vi "SmootherPath.vi"(6 "ball":T1, 8 "Robot in":T2={"id"=0, "function"=enum."Attacker", "x"=0.0, "y"=0.0, "orientation"=0.0, "v_tangent"=0.0, "v_normal"=0.0, "v_ang"=0.0, "kick_x"=0.0, "kick_z"=0.0, "dribble"=FALSE, "Timestamp"=timestamp(0 s since 1904-01-01), "estimatives"={"est_v_tangent"=0.0, "est_v_normal"=0.0, "est_vx"=0.0, "est_vy"=0.0, "Pos Robot Est"=[]}, "dest_x_kick"=0.0, "dest_y_kick"=0.0, "Gap Coord"=[], "States"=enum."GoToTangent", "Path "=[], "Path  Smooth"=[], "Dest"=[], "vx_desired"=0.0, "vy_desired"=0.0}, 9 "SmoothPath":dbl[][](array[numeric]), 10 "enemy_robots":T2[](array[typedef]), 11 "our_robots":T2[](array[typedef])) -> (1 "SmootherPath":dbl[][](array[numeric]))   [LabVIEW 2018]
uses:
  Vision_class/Old vision/Controls/AI Robot.ctl
  Vision_class/Old vision/Controls/Functions Enum.ctl
  Vision_class/Old vision/Controls/AttackerStates.ctl
  Vision_class/Old vision/Controls/PathDests.ctl
  Vision_class/Old vision/Controls/PathDest.ctl
  Communication_class/Paths/MessageAI_State Folder/Core/AI Ball.ctl
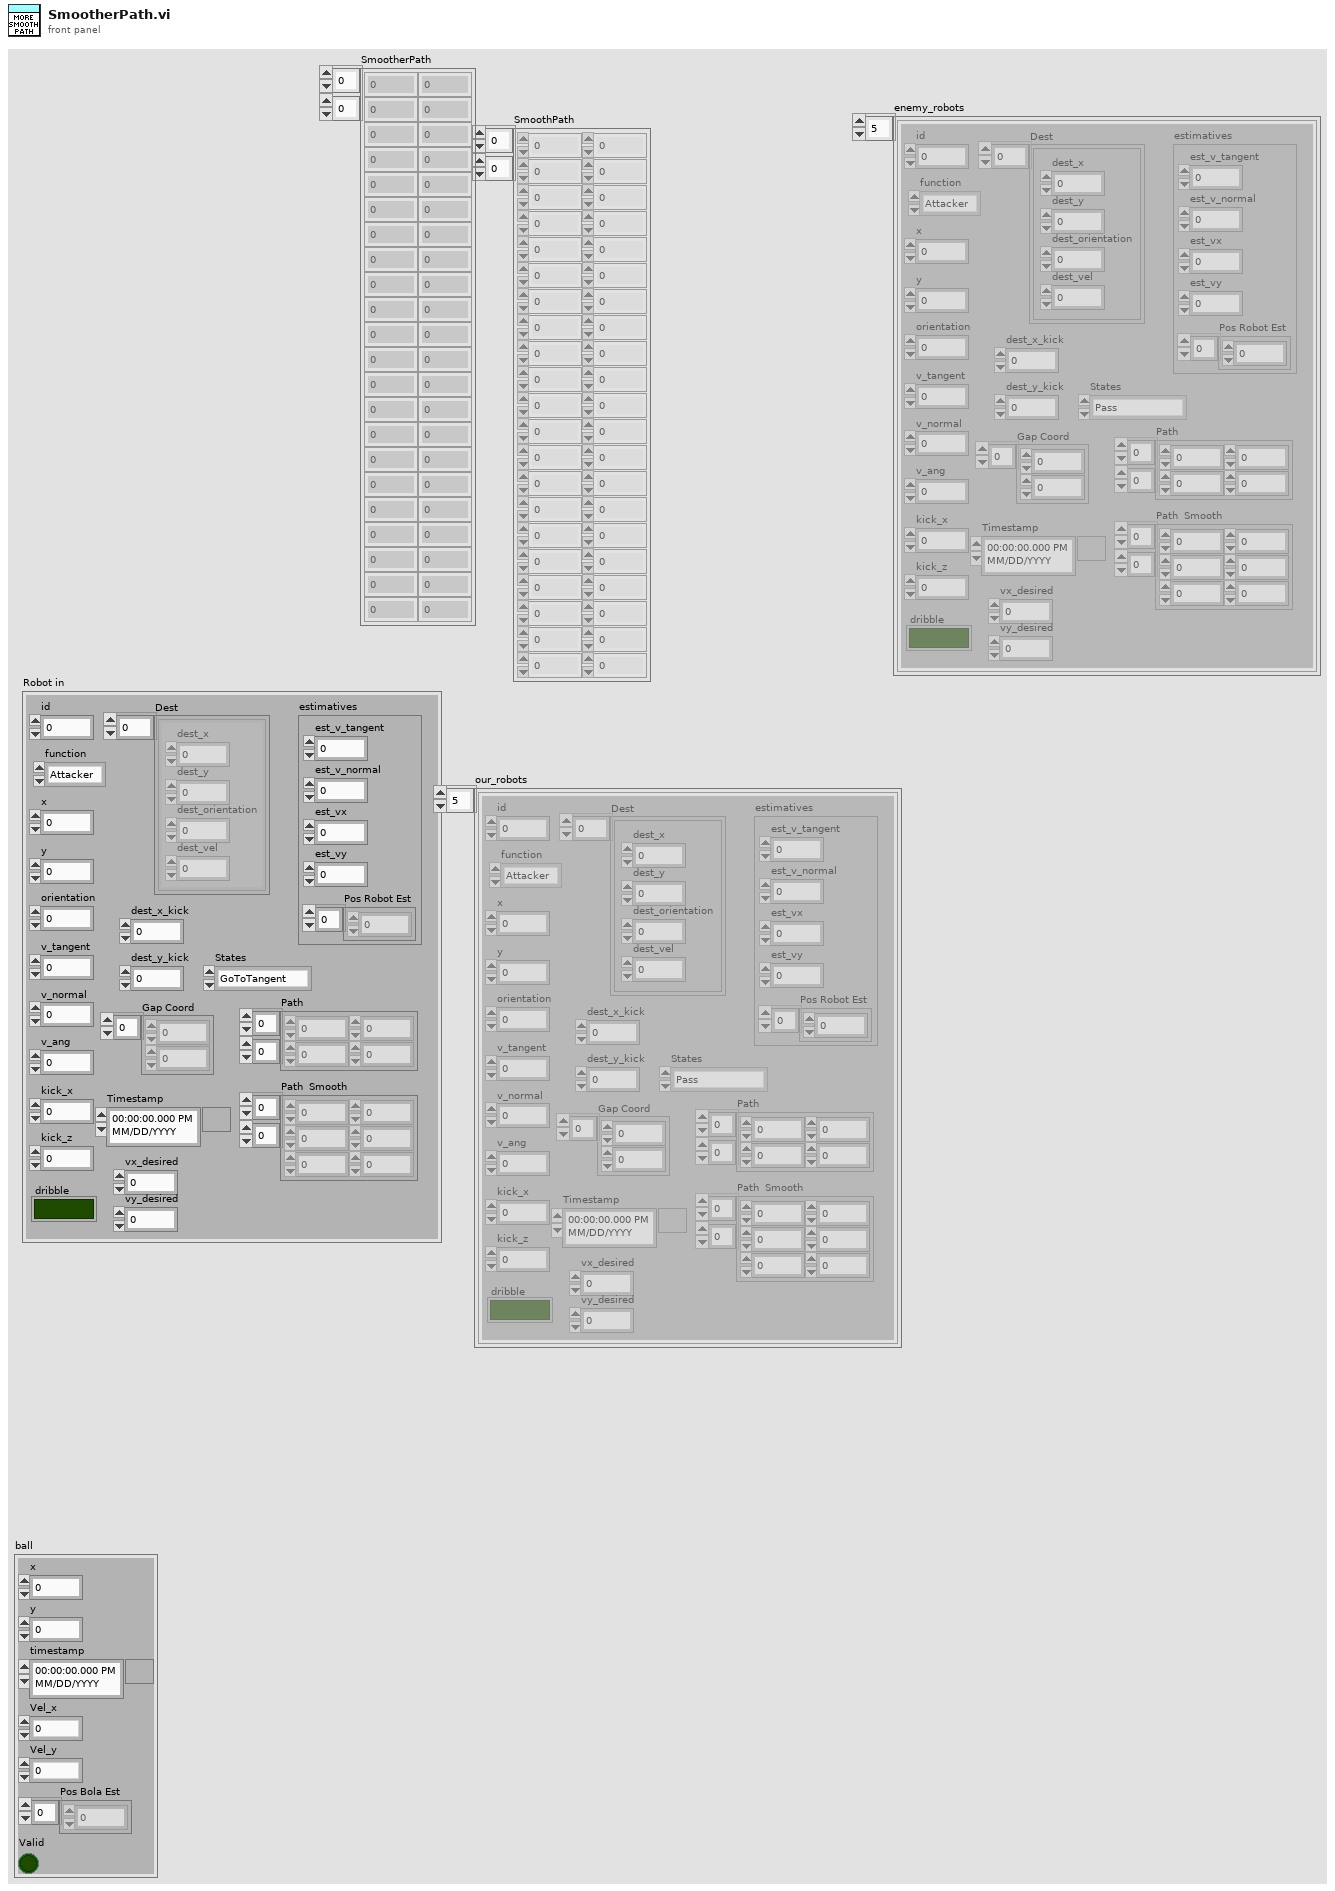
[diagram p1: front panel]
types:
  T1 = typedef "AI Ball.ctl" = cluster{"x":dbl, "y":dbl, "timestamp":timestamp, "Vel_x":dbl, "Vel_y":dbl, "Pos Bola Est":dbl[], "Valid":bool}
  T2 = typedef "AI Robot.ctl" = cluster{"id":u32, "function":T3, "x":dbl, "y":dbl, "orientation":dbl, "v_tangent":dbl, "v_normal":dbl, "v_ang":dbl, "kick_x":dbl, "kick_z":dbl, "dribble":bool, "Timestamp":timestamp, "estimatives":cluster{"est_v_tangent":dbl, "est_v_normal":dbl, "est_vx":dbl, "est_vy":dbl, "Pos Robot Est":dbl[]}, "dest_x_kick":dbl, "dest_y_kick":dbl, "Gap Coord":dbl[], "States":T4, "Path ":dbl[][], "Path  Smooth":dbl[][], "Dest":T5, "vx_desired":dbl, "vy_desired":dbl}
  T3 = typedef "Functions Enum.ctl" = enum16{"2nd Striker", "Attacker", "Goalie", "Defender", "Striker", "Goto 0", "Dummy", "Kicker", "ZigZag 0", "ZigZag 1", "ZigZag 2", "ZigZag 3", "ZigZag 4", "ZigZag 5", "ZigZag 6", "ZigZag 7", "ZigZag 8", ""}
  T4 = typedef "AttackerStates.ctl" = enum16{"Pass", "GoToTangent", "BallGetting", "GoToKick", ""}
  T5 = typedef "PathDests.ctl" = T6[]
  T6 = typedef "PathDest.ctl" = cluster{"dest_x":dbl, "dest_y":dbl, "dest_orientation":dbl, "dest_vel":dbl}
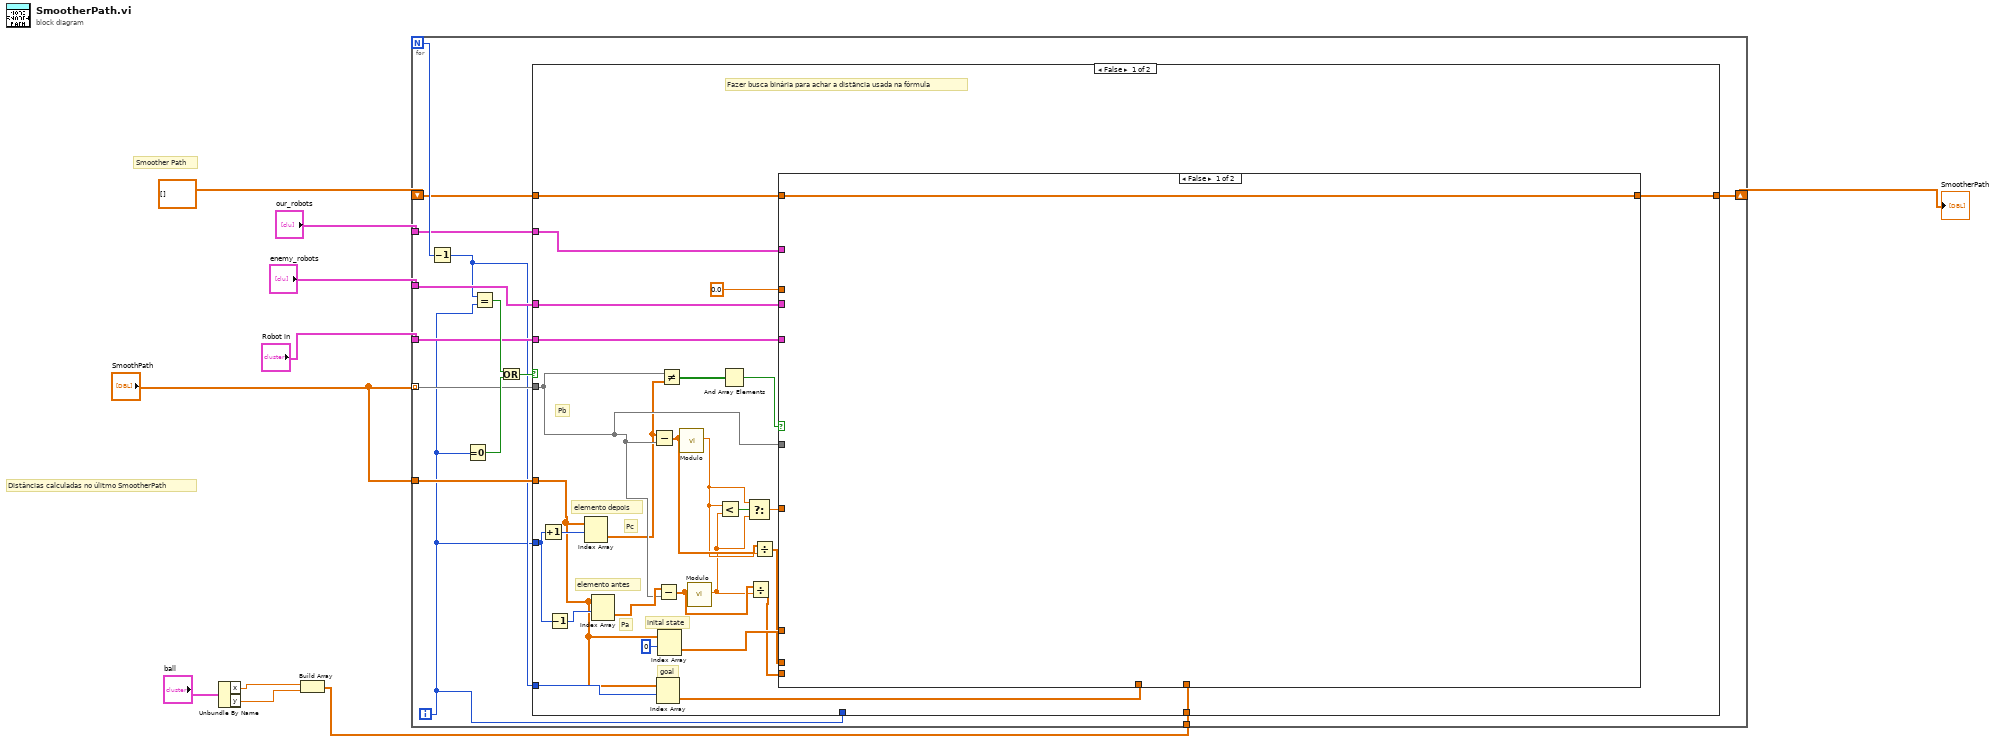
[diagram p0: block diagram]
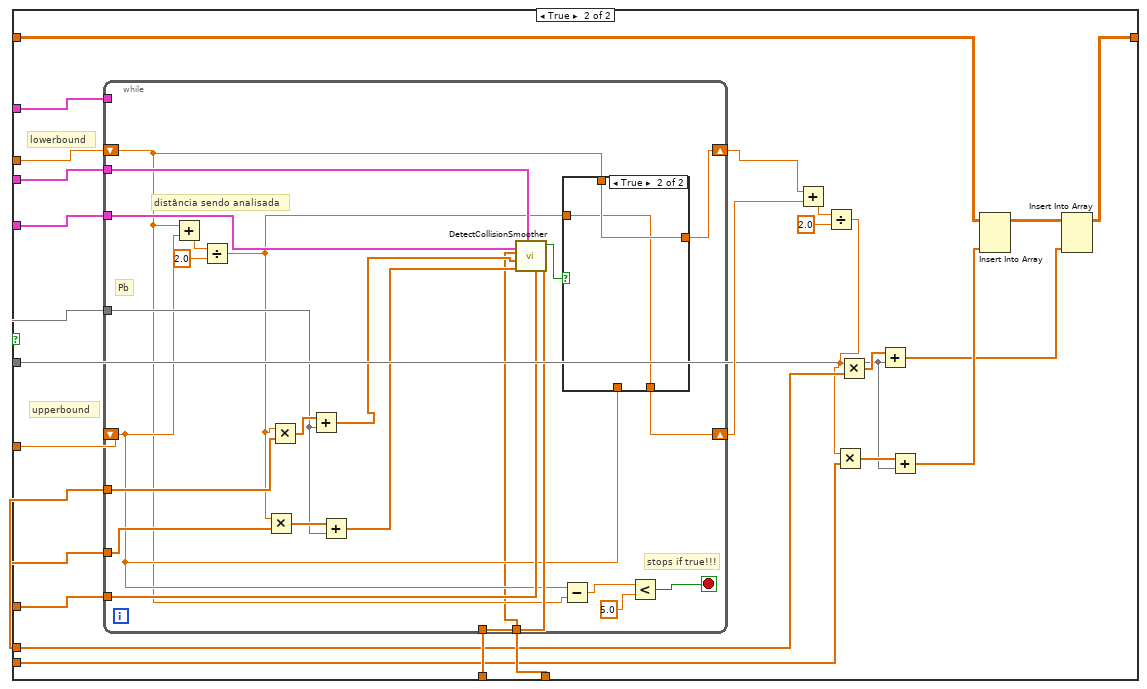
[diagram p2: hidden frame]
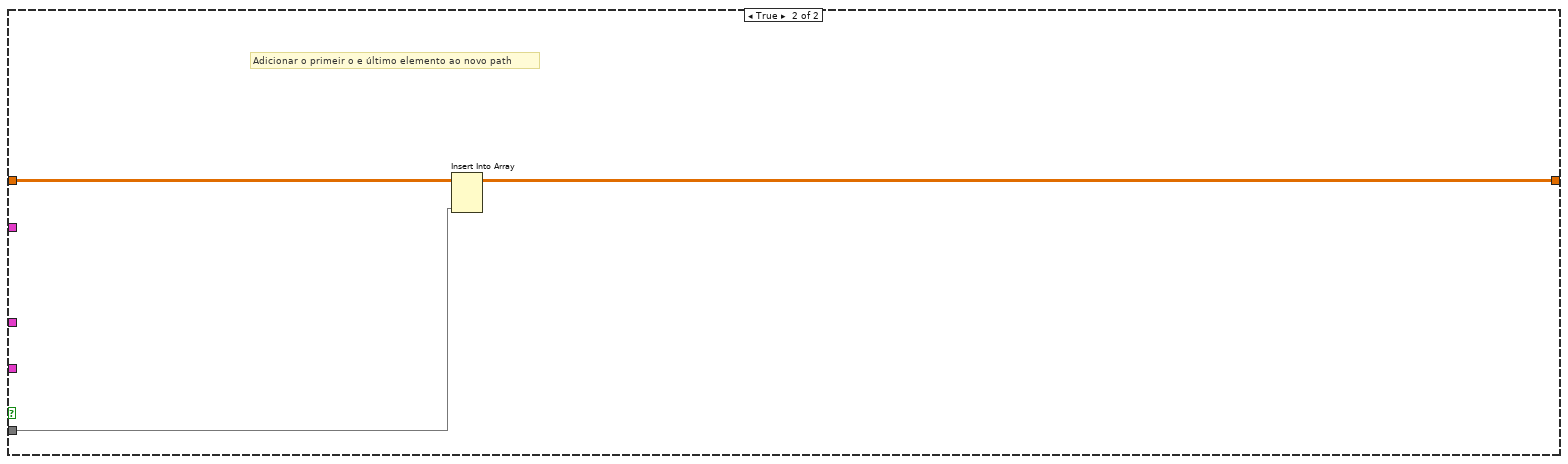
[diagram p4: hidden frame]
diagram:
  # "Distâncias calculadas no úlitmo SmootherPath"
  # "Smoother Path"
  n1 = Unbundle By Name("ball") -> ("x"=w9:dbl, "y"=w8:dbl)
  n2 = Build Array(w9, w8) -> (w3:dbl[])
  n3 = for {
    N -> [w24]
    tunnel: "SmoothPath" -> [w19] mode=indexing
    shift-right: [w18] -> w1
    shift-left: dbl[][] [] ("Path") -> [w21]
    tunnel: "SmoothPath" -> [w17]
    tunnel: "our_robots" -> [w16]
    tunnel: "enemy_robots" -> [w15]
    tunnel: "Robot in" -> [w14]
    tunnel: w3 -> [w12]
    i -> [w11]
    n4 = Decrement(x=w24) -> (x-1=w13:i32)
    n5 = Equal To 0?(x=w11) -> (x = 0?=w22:bool)
    n6 = Equal?(x=w13, y=w11) -> (x = y?=w23:bool)
    n7 = Or(x=w23, y=w22) -> (x .or. y?=w20:bool)
    n8 = case shown="False" w20 {
      tunnel: w21 -> [w34 w106]
      tunnel: w19 -> [w28 w105]
      tunnel: [w33 w104] -> w18
      tunnel: w17 -> [w29 _]
      tunnel: w11 -> [w31 _]
      tunnel: w16 -> [w43 _]
      tunnel: w15 -> [w42 _]
      tunnel: w14 -> [w41 _]
      tunnel: w13 -> [w39 _]
      tunnel: w12 -> [w36 _]
      tunnel: w11 -> [_ _]
      frame False {
        # "Pa"
        # "Pc"
        # "Pb"
        # "goal"
        # "inital state"
        # "elemento antes"
        # "elemento depois"
        # "Fazer busca binária para achar a distãncia usada na fórmula"
        n9 = Increment(x=w31) -> (x+1=w52:i32)
        n10 = Decrement(x=w31) -> (x-1=w51:i32)
        n11 = Index Array(array=w29, index (row)=w52) -> (element=w27:dbl[])  [unwired: 1 in]
        n12 = Index Array(array=w29, index (row)=w51) -> (element=w30:dbl[])  [unwired: 1 in]
        n13 = Subtract(x=w27, y=w28) -> (x-y=w47:dbl[])
        n14 = Index Array(array=w29, index (row)=w39) -> (element=w37:dbl[])  [unwired: 1 in]
        n15 = Subtract(x=w30, y=w28) -> (x-y=w45:dbl[])
        n16 = Index Array(array=w29, index (row)=0) -> (element=w38:dbl[])  [unwired: 1 in]
        n17 = Not Equal?(x=w28, y=w27) -> (x != y?=w26:bool[])
        n18 = call "Modulo.vi"("2D vector"=w47) -> ("Modulo"=w46:dbl)  [unwired: 10 in]
        n19 = call "Modulo.vi"("2D vector"=w45) -> ("Modulo"=w44:dbl)  [unwired: 10 in]
        n20 = Less?(x=w46, y=w44) -> (x < y?=w49:bool)
        n21 = And Array Elements(Boolean array=w26) -> (logical AND=w25:bool)
        n22 = Select(t=w46, s=w49, f=w44) -> (s? t:f=w48:dbl)
        n23 = Divide(x=w45, y=w44) -> (x/y=w32:dbl[])
        n24 = Divide(x=w47, y=w46) -> (x/y=w35:dbl[])
        n25 = case shown="False" w25 {
          tunnel: 0.0 -> [_ w76]
          tunnel: w48 -> [_ w75]
          tunnel: w43 -> [_ w74]
          tunnel: w42 -> [_ w73]
          tunnel: w41 -> [_ w72]
          tunnel: w38 -> [_ w71]
          tunnel: w37 -> [_ w70]
          tunnel: w36 -> [_ w69]
          tunnel: w35 -> [_ w62]
          tunnel: w34 -> [w53 w61]
          tunnel: [w53 w59] -> w33
          tunnel: w32 -> [_ w58]
          tunnel: w28 -> [_ w56]
          frame False {
          }
          frame True {
            # "upperbound"
            # "lowerbound"
            n26 = while {
              shift-right: [w82] -> w66
              shift-left: w76 -> [w80]
              shift-right: [w81] -> w65
              shift-left: w75 -> [w83]
              tunnel: w56 -> [w90]
              tunnel: w58 -> [w94]
              tunnel: w62 -> [w93]
              tunnel: w74 -> [_]
              tunnel: w73 -> [w89]
              tunnel: w72 -> [w88]
              tunnel: w71 -> [w87]
              tunnel: w70 -> [w86]
              tunnel: w69 -> [w77]
              stop <- w97 stop-if-true
              # "distância sendo analisada"
              # "Pb"
              # "stops if true!!!"
              n27 = Add(x=w80, y=w83) -> (x+y=w96:dbl)
              n28 = Divide(x=w96, y=2.0) -> (x/y=w84:dbl)
              n29 = Multiply(x=w84, y=w94) -> (x*y=w92:dbl[])
              n30 = Multiply(x=w84, y=w93) -> (x*y=w91:dbl[])
              n31 = Add(x=w91, y=w90) -> (x+y=w79:dbl[])
              n32 = Add(x=w92, y=w90) -> (x+y=w78:dbl[])
              n33 = call "DetectCollisionSmoother.vi"("Goal"=w86, "Initial State"=w87, "enemy_robots"=w89, "Robot in"=w88, "SegmentPointB"=w78, "SegmentPointA"=w79, "ball"=w77) -> ("Is there colision?"=w85:bool)  [unwired: 4 in]
              n34 = Subtract(x=w83, y=w80) -> (x-y=w99:dbl)
              n35 = case shown="True" w85 {
                tunnel: w84 -> [w101 w102]
                tunnel: w80 -> [_ w103]
                tunnel: w83 -> [w100 _]
                tunnel: [w101 w103] -> w82
                tunnel: [w100 w102] -> w81
                frame False {
                }
                frame True {
                }
              }
              n36 = Less?(x=w99, y=5.0) -> (x < y?=w97:bool)
            }
            n37 = Add(x=w66, y=w65) -> (x+y=w68:dbl)
            n38 = Divide(x=w68, y=2.0) -> (x/y=w57:dbl)
            n39 = Multiply(x=w57, y=w58) -> (x*y=w64:dbl[])
            n40 = Multiply(x=w57, y=w62) -> (x*y=w63:dbl[])
            n41 = Add(x=w63, y=w56) -> (x+y=w54:dbl[])
            n42 = Add(x=w64, y=w56) -> (x+y=w55:dbl[])
            n43 = Insert Into Array(array=w61, new element=w55) -> (w60:dbl[][])  [unwired: 2 in]
            n44 = Insert Into Array(array=w60, new element=w54) -> (w59:dbl[][])  [unwired: 2 in]
          }
        }
      }
      frame True {
        # "Adicionar o primeir o e último elemento ao novo path"
        n45 = Insert Into Array(array=w106, new element=w105) -> (w104:dbl[][])  [unwired: 2 in]
      }
    }
  }
  "SmootherPath" <- w1
